vi "Find Node Error Terminal.vi"(8 "error in (no erros)":errorcluster, 10 "source/sink":enum16{"Source", "Sink"}(ring), 11 "diagram in":refnum<vi>) -> (0 "error out":errorcluster, 2 "error terminal":refnum<vi>, 3 "diagram out":refnum<vi>)   [LabVIEW 2017]
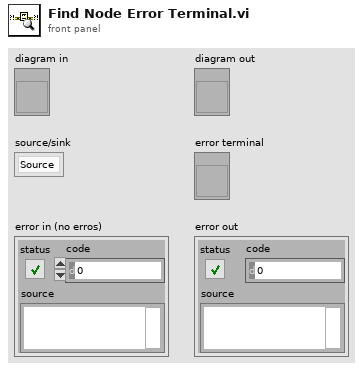
[diagram p1: front panel]
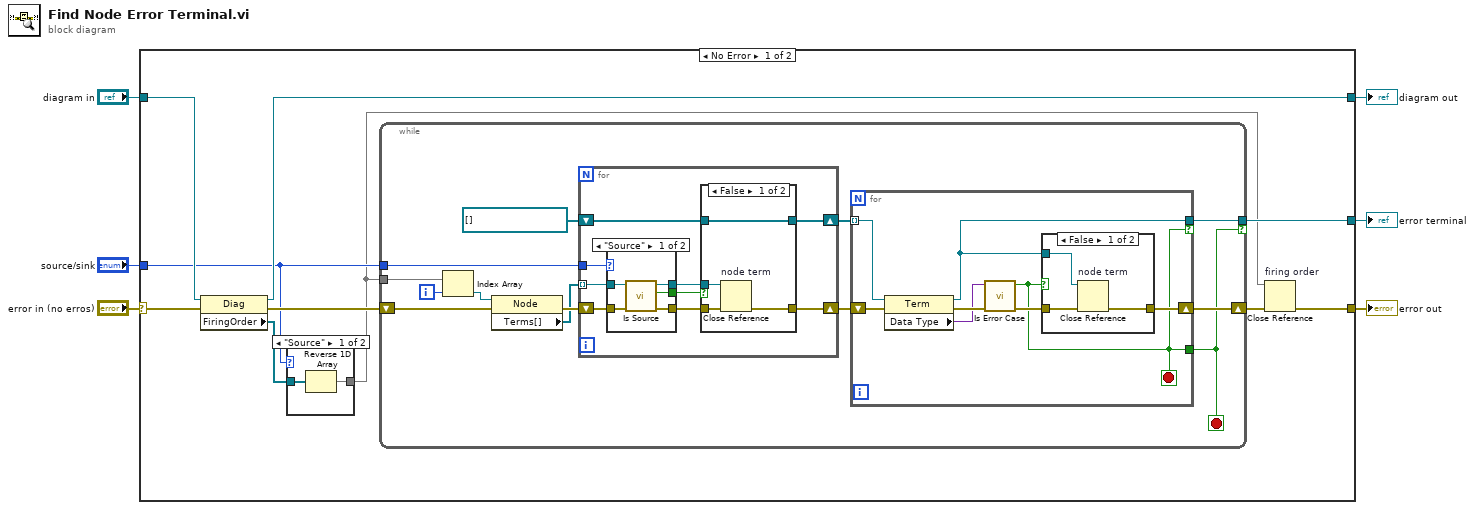
[diagram p0: block diagram]
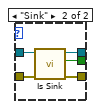
[diagram p3: hidden frame]
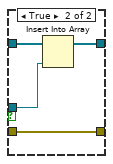
[diagram p4: hidden frame]
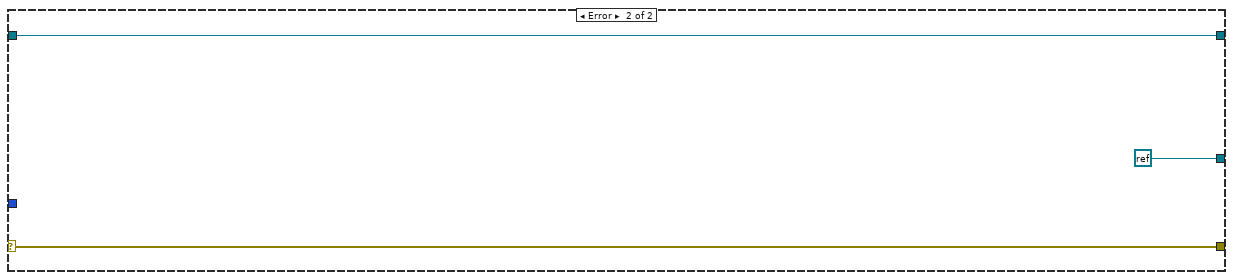
[diagram p6: hidden frame]
diagram:
  n1 = case shown="No Error" "error in (no erros)" {
    selector: "error in (no erros)" -> [w7 w73]
    tunnel: [w16 refnum<k0> refnum] -> w6
    tunnel: [w14 w73] -> w5
    tunnel: "diagram in" -> [w12 w74]
    tunnel: [w11 w74] -> w3
    tunnel: "source/sink" -> [w10 _]
    frame No Error {
      n2 = property class="Diag"(reference=w12, error in=w7) -> (reference out=w11:refnum<vi>, error out=w13:errorcluster, "FiringOrder"=w9:refnum<vi>[])
      n3 = case shown="\"Source\"" w10 {
        tunnel: [w17 w19] -> w8
        tunnel: w9 -> [w18 w19]
        frame "Source" {
          n4 = Reverse 1D Array(array=w18) -> (reversed array=w17:refnum<vi>[])
        }
        frame "Sink" {
        }
      }
      n5 = while {
        shift-right: [w31] -> w15
        shift-left: w13 -> [w25]
        tunnel: [w30] -> w16 if=w29
        tunnel: w8 -> [w27]
        tunnel: w10 -> [w21]
        i -> [w26]
        stop <- w29 stop-if-true
        n6 = Index Array(array=w27, index=w26) -> (element=w24:refnum<vi>)
        n7 = property class="Node"(reference=w24, error in=w25) -> (error out=w32:errorcluster, "Terms[]"=w28:refnum<vi>[])  [unwired: 1 out]
        n8 = for {
          tunnel: w28 -> [w41] mode=indexing
          shift-right: [w38] -> w20
          shift-left: w32 -> [w37]
          shift-right: [w36] -> w22
          shift-left: refnum<vi>[] [] -> [w35]
          tunnel: w21 -> [w34]
          n9 = case shown="\"Source\"" w34 {
            tunnel: w41 -> [w46 w51]
            tunnel: [w44 w50] -> w40
            tunnel: [w43 w47] -> w39
            tunnel: w37 -> [w45 w48]
            tunnel: [w42 w49] -> w33
            frame "Source" {
              n10 = call "Is Source.vi"("error in (no error)"=w45, "terminal in"=w46) -> ("error out"=w43:errorcluster, "is source"=w42:bool, "terminal out"=w44:refnum<vi>)  [unwired: 7 in]
            }
            frame "Sink" {
              n11 = call "Is Sink.vi"("error in (no error)"=w48, "terminal in"=w51) -> ("error out"=w47:errorcluster, "is sink?"=w49:bool, "terminal out"=w50:refnum<vi>)  [unwired: 7 in]
            }
          }
          n12 = case shown="False" w33 {
            tunnel: w40 -> [w55 w58]
            tunnel: w39 -> [w54 w59]
            tunnel: [w53 w59] -> w38
            tunnel: [w52 w57] -> w36
            tunnel: w35 -> [w52 w56]
            frame False {
              n13 = Close Reference "node term"(reference=w55, error in (no error)=w54) -> (error out=w53:errorcluster)
            }
            frame True {
              n14 = Insert Into Array(array=w56, new element=w58) -> (w57:refnum<vi>[])  [unwired: 1 in]
            }
          }
        }
        n15 = for {
          tunnel: w22 -> [w66] mode=indexing
          shift-right: [w64] -> w31
          shift-left: w20 -> [w65]
          tunnel: [w63] -> w30 if=w60
          tunnel: [w60] -> w29
          stop <- w60 stop-if-true
          n16 = property class="Term"(reference=w66, error in=w65) -> (reference out=w63:refnum<vi>, error out=w67:errorcluster, "Data Type"=w62:variant)
          n17 = call "Is Error Case.vi"("error in (no error)"=w67, "variant"=w62) -> ("error out"=w61:errorcluster, "error cluster?"=w60:bool)  [unwired: 8 in]
          n18 = case shown="False" w60 {
            tunnel: [w70 w71] -> w64
            tunnel: w63 -> [w69 _]
            tunnel: w61 -> [w68 w71]
            frame False {
              n19 = Close Reference "node term"(reference=w69, error in (no error)=w68) -> (error out=w70:errorcluster)
            }
            frame True {
            }
          }
        }
      }
      n20 = Close Reference "firing order"(reference=w8, error in (no error)=w15) -> (error out=w14:errorcluster)
    }
    frame Error {
    }
  }
  "error terminal" <- w6
  "error out" <- w5
  "diagram out" <- w3
